vi "Configure Wiring.vi"(0 "VISA resource name":refnum<visa-resource-name>, 1 "Wiring C (1: 1p2W)":u16(ring)=1 items=["NONE", "1P2W", "1P3W", "3P3W", "3P4W", "3P3W(3V3A)"], 2 "Wiring B (1: 1p2W)":u16(ring)=1 items=["NONE", "1P2W", "1P3W", "3P3W", "3P4W", "3P3W(3V3A)"], 3 "Wiring A (1: 1p2W)":u16(ring)=1 items=["1P2W"=1, "1P3W"=2, "3P3W"=3, "3P4W"=4, "3P3W(3V3A)"=5], 5 "Wiring D (1: 1p2W)":u16(ring)=1 items=["NONE", "1P2W", "1P3W", "3P3W", "3P4W", "3P3W(3V3A)"], 7 "Wiring E (1: 1p2W)":u16(ring)=1 items=["NONE", "1P2W", "1P3W", "3P3W"], 9 "Wiring F (1: 1p2W)":u16(ring)=1 items=["NONE", "1P2W"], 11 "error in (no error)":errorcluster) -> (4 "VISA resource name out":refnum<visa-resource-name>, 15 "error out":errorcluster)   [LabVIEW 2021, in "Yokogawa WT1800 Series.lvlib"]
doc: "Sets the wiring system."
uses:
  <instrlib>/Yokogawa WT1800 Series/Yokogawa WT1800 Series.lvlib
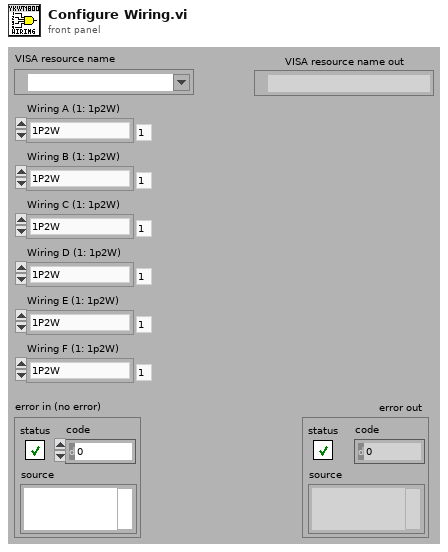
[diagram p1: front panel]
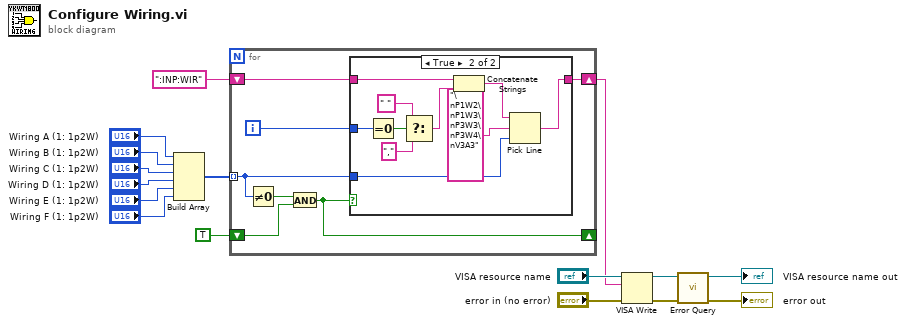
[diagram p0: block diagram]
diagram:
  n1 = Build Array("Wiring A (1: 1p2W)", "Wiring B (1: 1p2W)", "Wiring C (1: 1p2W)", "Wiring D (1: 1p2W)", "Wiring E (1: 1p2W)", "Wiring F (1: 1p2W)") -> (w4:u16[])
  n2 = for {
    tunnel: w4 -> [w17] mode=indexing
    shift-right: [w22] -> w1
    shift-left: ":INP:WIR" -> [w23]
    shift-right: [w19] -> _
    shift-left: TRUE -> [w18]
    i -> [w21]
    n3 = Not Equal To 0?(x=w17) -> (x != 0?=w20:bool)
    n4 = And(x=w20, y=w18) -> (x .and. y?=w19:bool)
    n5 = case shown="True" w19 {
      tunnel: w23 -> [w24 w28]
      tunnel: [w24 w33] -> w22
      tunnel: w21 -> [_ w31]
      tunnel: w17 -> [_ w25]
      frame False {
      }
      frame True {
        n6 = Equal To 0?(x=w31) -> (x = 0?=w32:bool)
        n7 = Select(t=" ", s=w32, f=",") -> (s? t:f=w27:string)
        n8 = Concatenate Strings(w28, w27) -> (w26:string)
        n9 = Pick Line ("ライン選択")(string ("")=w26, multi-line string="\nP1W2\nP1W3\nP3W3\nP3W4\nV3A3", line index=w25) -> (output string=w33:string)
      }
    }
  }
  n10 = VISA Write ("VISA書き込み")(VISA resource name="VISA resource name", write buffer=w1, error in (no error)="error in (no error)") -> (VISA resource name out=w12:refnum<visa-resource-name>, error out=w11:errorcluster)  [unwired: 1 out]
  n11 = call <instrlib>:"Error Query.vi"("error in (no error)"=w11, "VISA resource name"=w12) -> ("error out"=→"error out":errorcluster, "VISA resource name out"=→"VISA resource name out":refnum<visa-resource-name>)  [unwired: 6 in, 2 out]
